vi "DifferentialVoltage Setter.vi"(0 "LimitReverseMotion":bool, 1 "EnableFOC":bool=TRUE, 2 "OverrideBrakeDurNeutral":bool, 3 "Update Frequency (Hz)":dbl=100.0, 5 "StopSendingOtherRequests":bool=TRUE, 7 "TargetOutput":dbl, 9 "DifferentialPosition":dbl, 12 "DifferentialSlot":i32=1, 13 "LimitForwardMotion":bool) -> (4 "DeviceReference Out":T1)   [LabVIEW 2023]
doc: "Request a specified voltage with a differential position closed-loop.\nThis control mode will attempt to apply the specified voltage to the motor. If the supply voltage is below the requested voltage, the motor controller will output the supply voltage. It will also set the motor's differential position setpoint to the specified position."
uses:
  Users/Cory/Documents/PhoenixPro-LabVIEW-Generation/controls/DeviceReference.ctl
panel:
  in  "DeviceReference":T1
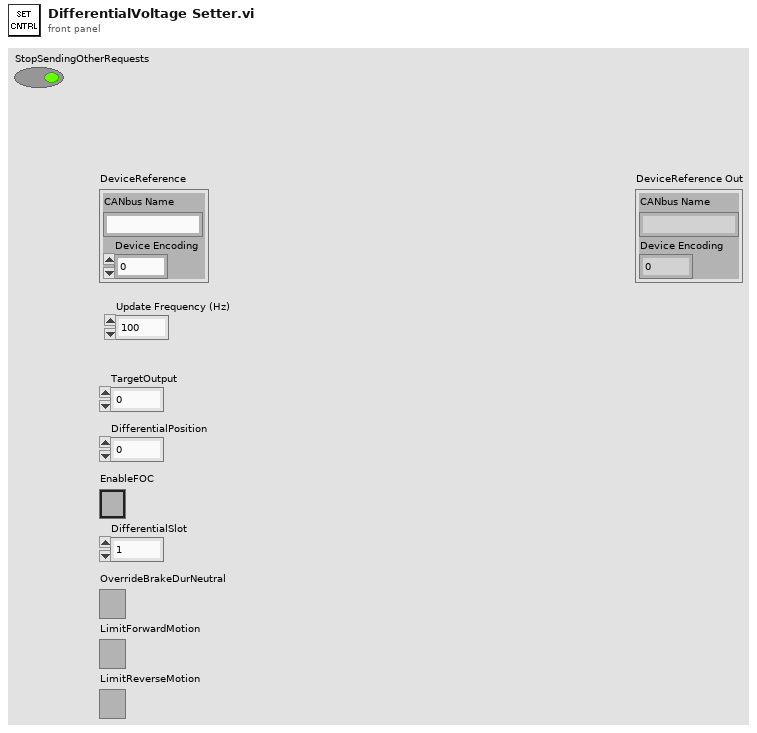
[diagram p1: front panel]
types:
  T1 = typedef "DeviceReference.ctl" = cluster{"CANbus Name":string, "Device Encoding":u32}
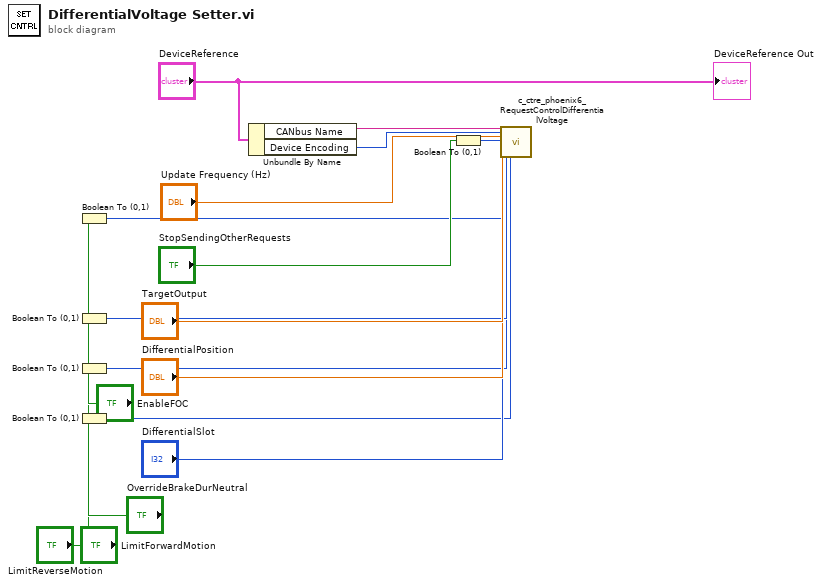
[diagram p0: block diagram]
diagram:
  n1 = Boolean To (0,1)(Boolean="EnableFOC") -> (0, 1=w8:i16)
  n2 = Boolean To (0,1)(Boolean="OverrideBrakeDurNeutral") -> (0, 1=w5:i16)
  n3 = Boolean To (0,1)(Boolean="LimitForwardMotion") -> (0, 1=w3:i16)
  n4 = Boolean To (0,1)(Boolean="LimitReverseMotion") -> (0, 1=w1:i16)
  n5 = Unbundle By Name("DeviceReference") -> ("CANbus Name"=w16:string, "Device Encoding"=w15:u32)
  n6 = Boolean To (0,1)(Boolean="StopSendingOtherRequests") -> (0, 1=w12:i16)
  n7 = call <vilib>:"c_ctre_phoenix6_RequestControlDifferentialVoltage.vi"("String"=w16, "Numeric 2"=w15, "Numeric 3"="Update Frequency (Hz)", "Numeric 4"=w12, "Numeric 5"="TargetOutput", "Numeric 6"="DifferentialPosition", "Numeric 7"=w8, "Numeric 8"="DifferentialSlot", "Numeric 9"=w5, "Numeric 10"=w3, "Numeric 11"=w1) -> ()  [unwired: 16 in, 1 out]
  "DeviceReference Out" <- "DeviceReference"
